vi "PH_Sequencer.PC Switch Seq SM.vi"(0 "i ref in":refnum<vi>, 5 "error IO":errorcluster) -> (14 "i ref out":refnum<vi>, 19 "error out":errorcluster)   [LabVIEW 2014, in "PH_Sequencer.lvlib"]
uses:
  PH_Sequencer.lvlib
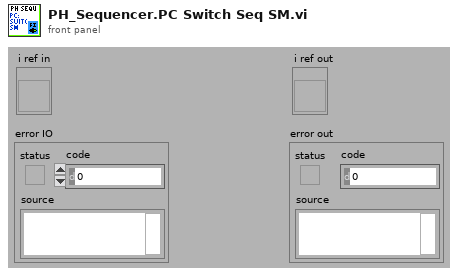
[diagram p1: front panel]
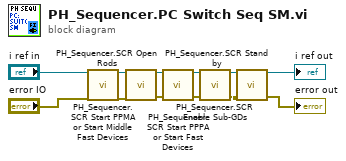
[diagram p0: block diagram]
diagram:
  n1 = call "PH_Sequencer.SCR Start PPMA or Start Middle Fast Devices.vi"("i ref in"="i ref in", "error in (no error)"="error IO") -> ("i ref out"=w3:refnum<vi>, "error out"=w4:errorcluster)  [unwired: 16 in]
  n2 = call "PH_Sequencer.SCR Open Rods.vi"("i ref in"=w3, "error in (no error)"=w4) -> ("i ref out"=w5:refnum<vi>, "error out"=w6:errorcluster)  [unwired: 16 in]
  n3 = call "PH_Sequencer.SCR Start PPPA or Start Fast Devices.vi"("i ref in"=w5, "error in (no error)"=w6) -> ("i ref out"=w7:refnum<vi>, "error out"=w8:errorcluster)  [unwired: 16 in]
  n4 = call "PH_Sequencer.SCR Enable Sub-GDs.vi"("i ref in"=w7, "error in (no error)"=w8) -> ("i ref out"=w9:refnum<vi>, "error out"=w10:errorcluster)  [unwired: 16 in]
  n5 = call "PH_Sequencer.SCR Stand by.vi"("i ref in"=w9, "error in (no error)"=w10) -> ("i ref out"=→"i ref out":refnum<vi>, "error out"=→"error out":errorcluster)  [unwired: 16 in]
